vi "Stream LLP Packets to Disk New.vi"(0 "fpga interface in":refnum<k20>, 1 "bytes acquired indicator ref":refnum<vi>, 5 "serial input channel":string, 7 "base packet file path":path, 9 "fetch size (elements)":u32=40960, 11 "error in (no error)":errorcluster, 12 "fetch timeout (s)":dbl=1.0, 13 "log to disk":bool=TRUE) -> (4 "fpga interface out":refnum<k20>, 6 "file path out":path, 8 "acquisition error":bool, 15 "error out":errorcluster)   [LabVIEW 2026]
uses:
  Types/148x_Acq_FPGA_Reference.ctl
  0829f115-c11d-4785-86b3-38f743f517d6.vi
  <vilib>/rvi/errors/niLvFpgaAdjustHostInterfaceError.vi
  <vilib>/rvi/interface/nirviMethod/nirviMethod.xnode
  <vilib>/rvi/interface/nirviReadWriteControl/nirviReadWriteControl.xnode
  <vilib>/FPGAPlugInAG/Dynamic/niLvFpga_AcquireReadRegionFifo_Dynamic.vi
  <vilib>/rvi/errors/niLvFpgaMergeErrorWithErrorCode.vi
  <instrlib>/FlexRIO/Automotive Vision Utility/v1/Host/Automotive Vision Utility.lvlib
  GettingStarted_Acq_148X_Host.lvlib
  Common/GettingStarted_Common_148X_Host.lvlib
  NiFpgaLv.dll
  <vilib>/rvi/interface/Simulation/niFpgaSimulationCallBeginRW.vi
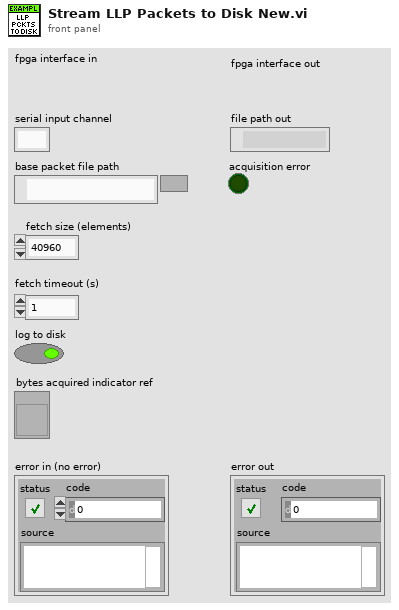
[diagram p1: front panel]
types:
  T1 = typedef "Automotive Vision Utility.lvlib/Serial Channel Type.ctl" = enum16{"Serial Input Channel", "Serial Output Channel", "Unknown Channel Type"}
  T2 = typedef "GettingStarted_Acq_148X_Host.lvlib/148x_Acq_FPGA_Reference.ctl" = refnum<k20>
  T3 = cluster{"acq state":enum8{"Idle", "Wait for First Packet Header", "Acquire", "Wait for Last Packet Header", "Wait for End of Last Packet"}, "stop timed out":bool, "bad packet header":bool, "bad packet payload":bool, "bad packet size":bool, "dram status":cluster{"bytes written":u64, "bytes read":u64, "overflow":bool, "partition full":bool, "last byte flushed":bool}}[]
  T4 = cluster{"acq state":enum8{"Idle", "Wait for First Packet Header", "Acquire", "Wait for Last Packet Header", "Wait for End of Last Packet"}, "stop timed out":bool, "bad packet header":bool, "bad packet payload":bool, "bad packet size":bool, "dram status":cluster{"bytes written":u64, "bytes read":u64, "overflow":bool, "partition full":bool, "last byte flushed":bool}}
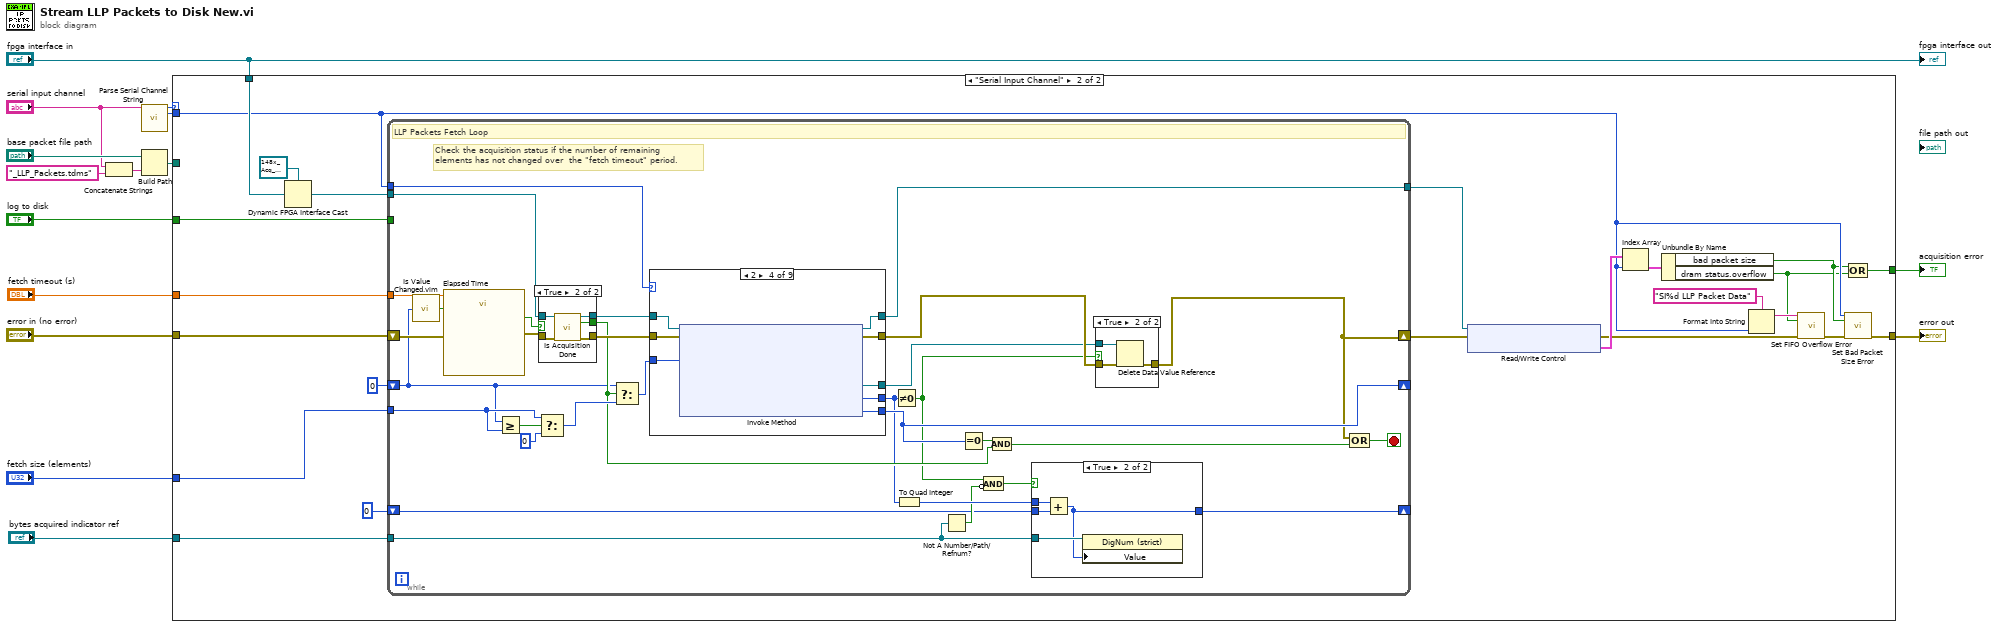
[diagram p0: block diagram]
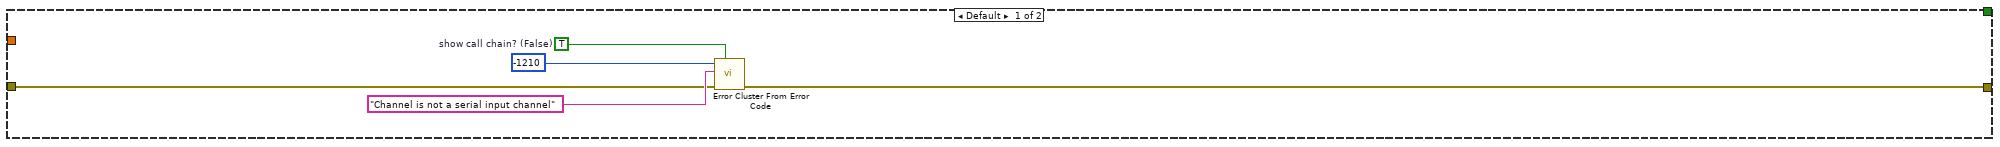
[diagram p2: hidden frame]
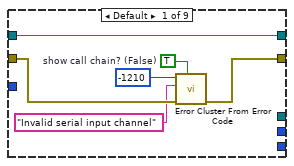
[diagram p6: hidden frame]
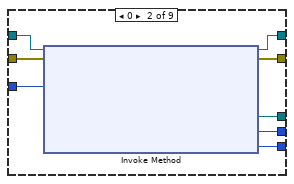
[diagram p7: hidden frame]
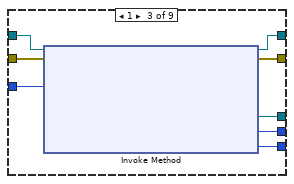
[diagram p8: hidden frame]
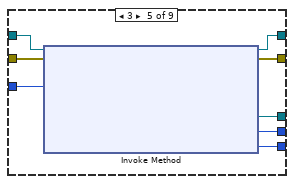
[diagram p9: hidden frame]
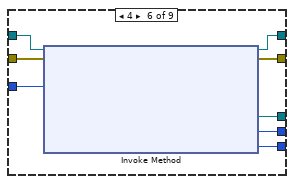
[diagram p10: hidden frame]
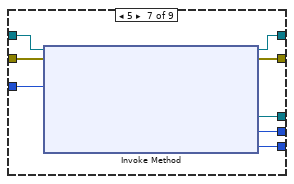
[diagram p11: hidden frame]
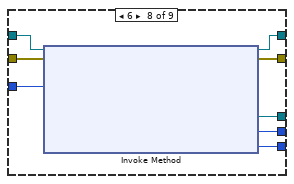
[diagram p12: hidden frame]
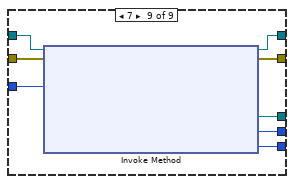
[diagram p13: hidden frame]
diagram:
  n1 = Concatenate Strings("serial input channel", "_LLP_Packets.tdms") -> (w8:string)
  n2 = call <instrlib>:"Parse Serial Channel String.vi"("serial channel string"="serial input channel") -> ("serial channel type"=w11:T1, "channel number"=w12:i32)  [unwired: 13 in]
  n3 = Build Path(base path="base packet file path", name or relative path=w8) -> (appended path=w5:path)
  n4 = case shown="\"Serial Input Channel\"" w11 {
    tunnel: "error in (no error)" -> [w17 w43]
    tunnel: w5 -> [_ _]
    tunnel: [w16 w25] -> w14
    tunnel: [_ w21] -> w13
    tunnel: w12 -> [_ w24]
    tunnel: "fetch size (elements)" -> [_ w40]
    tunnel: "fpga interface in" -> [_ w39]
    tunnel: "fetch timeout (s)" -> [_ w36]
    tunnel: "log to disk" -> [_ w29]
    tunnel: "bytes acquired indicator ref" -> [_ w27]
    frame Default {
      w18 = TRUE  # show call chain? (False)
      n5 = call <vilib>:"Error Cluster From Error Code.vi"("show call chain? (False)"=w18, "error in (no error)"=w17, "error message (\"\")"="Channel is not a serial input channel" ("error message (\"\")"), "error code (0)"=-1210) -> ("error out"=w16:errorcluster)  [unwired: 5 in]
    }
    frame "Serial Input Channel" {
      n6 = Dynamic FPGA Interface Cast(Session In=T2 refnum ("FPGA VI Reference Out"), Type=w39) -> (Session Out=w37:T2)
      n7 = while {
        shift-right: [w54] -> w35
        shift-left: w43 -> [w59]
        tunnel: w37 -> [w63]
        shift-right: [w55] -> _
        shift-left: u32 0 ("Elements Remaining") -> [w56]
        tunnel: [w71] -> w34
        tunnel: w24 -> [w74]
        tunnel: w40 -> [w65]
        tunnel: w36 -> [w70]
        tunnel: w29 -> [_]
        shift-right: [w46] -> _
        shift-left: i64 0 -> [w45]
        tunnel: w27 -> [w47]
        stop <- w75 stop-if-true
        # "Check the acquisition status if the number of remaining \nelements has not changed over  the \"fetch timeout\" period."
        # "LLP Packets Fetch Loop"
        n8 = call "Is Value Changed.vim"("value"=w56) -> ("changed or first call?"=w69:bool)
        n9 = call "Elapsed Time"("Time Target (s)"=w70, "Reset"=w69, "error in (no error)"=w59) -> ("Time has Elapsed"=w61:bool, "error out"=w58:errorcluster)  [unwired: 9 in, 6 out]
        n10 = Greater Or Equal?(x=w56, y=w65) -> (x >= y?=w68:bool)
        n11 = case shown="True" w61 {
          tunnel: w58 -> [w86 w91]
          tunnel: [w86 w90] -> w64
          tunnel: w63 -> [w85 w89]
          tunnel: [w85 w88] -> w62
          tunnel: [_ w87] -> w60
          frame False {
          }
          frame True {
            n12 = call "Is Acquisition Done.vi"("fpga interface in"=w89, "error in (no error)"=w91) -> ("fpga interface out"=w88:T2, "acquisition done"=w87:bool, "error out"=w90:errorcluster)  [unwired: 11 in]
          }
        }
        n13 = Select(t=w65, s=w68, f=u32 0 ("Elements Remaining")) -> (s? t:f=w66:u32)
        n14 = Select(t=w56, s=w60, f=w66) -> (s? t:f=w67:u32)
        n15 = case shown="2" w74 {
          tunnel: w62 -> [w97 w105 w113 w121 w129 w137 w145 w153 w161]
          tunnel: w64 -> [w96 w104 w112 w120 w128 w136 w144 w152 w160]
          tunnel: [_ w103 w111 w119 w127 w135 w143 w151 w159] -> w52
          tunnel: [_ w102 w110 w118 w126 w134 w142 w150 w158] -> w44
          tunnel: w67 -> [_ w101 w109 w117 w125 w133 w141 w149 w157]
          tunnel: [w93 w99 w107 w115 w123 w131 w139 w147 w155] -> w53
          tunnel: [_ w100 w108 w116 w124 w132 w140 w148 w156] -> w55
          tunnel: [w97 w98 w106 w114 w122 w130 w138 w146 w154] -> w71
          frame Default {
            w92 = TRUE  # show call chain? (False)
            n16 = call <vilib>:"Error Cluster From Error Code.vi"("show call chain? (False)"=w92, "error in (no error)"=w96, "error message (\"\")"="Invalid serial input channel" ("error message (\"\")"), "error code (0)"=-1210) -> ("error out"=w93:errorcluster)  [unwired: 5 in]
          }
          frame 0 {
            n17 = xnode "Invoke Method"("FPGA VI Reference In"=w105, "error in"=w104, "Number of Elements"=w101) -> ("FPGA VI Reference Out"=w98:T2, "error out"=w99:errorcluster, "Read Region Reference"=w103:refnum<data-value>, "Elements In Region"=w102:u32, "Elements Remaining"=w100:u32)  [unwired: 1 in]
          }
          frame 1 {
            n18 = xnode "Invoke Method"("FPGA VI Reference In"=w113, "error in"=w112, "Number of Elements"=w109) -> ("FPGA VI Reference Out"=w106:T2, "error out"=w107:errorcluster, "Read Region Reference"=w111:refnum<data-value>, "Elements In Region"=w110:u32, "Elements Remaining"=w108:u32)  [unwired: 1 in]
          }
          frame 2 {
            n19 = xnode "Invoke Method"("FPGA VI Reference In"=w121, "error in"=w120, "Number of Elements"=w117) -> ("FPGA VI Reference Out"=w114:T2, "error out"=w115:errorcluster, "Read Region Reference"=w119:refnum<data-value>, "Elements In Region"=w118:u32, "Elements Remaining"=w116:u32)  [unwired: 1 in]
          }
          frame 3 {
            n20 = xnode "Invoke Method"("FPGA VI Reference In"=w129, "error in"=w128, "Number of Elements"=w125) -> ("FPGA VI Reference Out"=w122:T2, "error out"=w123:errorcluster, "Read Region Reference"=w127:refnum<data-value>, "Elements In Region"=w126:u32, "Elements Remaining"=w124:u32)  [unwired: 1 in]
          }
          frame 4 {
            n21 = xnode "Invoke Method"("FPGA VI Reference In"=w137, "error in"=w136, "Number of Elements"=w133) -> ("FPGA VI Reference Out"=w130:T2, "error out"=w131:errorcluster, "Read Region Reference"=w135:refnum<data-value>, "Elements In Region"=w134:u32, "Elements Remaining"=w132:u32)  [unwired: 1 in]
          }
          frame 5 {
            n22 = xnode "Invoke Method"("FPGA VI Reference In"=w145, "error in"=w144, "Number of Elements"=w141) -> ("FPGA VI Reference Out"=w138:T2, "error out"=w139:errorcluster, "Read Region Reference"=w143:refnum<data-value>, "Elements In Region"=w142:u32, "Elements Remaining"=w140:u32)  [unwired: 1 in]
          }
          frame 6 {
            n23 = xnode "Invoke Method"("FPGA VI Reference In"=w153, "error in"=w152, "Number of Elements"=w149) -> ("FPGA VI Reference Out"=w146:T2, "error out"=w147:errorcluster, "Read Region Reference"=w151:refnum<data-value>, "Elements In Region"=w150:u32, "Elements Remaining"=w148:u32)  [unwired: 1 in]
          }
          frame 7 {
            n24 = xnode "Invoke Method"("FPGA VI Reference In"=w161, "error in"=w160, "Number of Elements"=w157) -> ("FPGA VI Reference Out"=w154:T2, "error out"=w155:errorcluster, "Read Region Reference"=w159:refnum<data-value>, "Elements In Region"=w158:u32, "Elements Remaining"=w156:u32)  [unwired: 1 in]
          }
        }
        n25 = Not Equal To 0?(x=w44) -> (x != 0?=w48:bool)
        n26 = To Quad Integer(1:w44) -> (0:w51:i64)
        n27 = Not A Number/Path/Refnum?(number/path/refnum=w47) -> (NaN/Path/Refnum?=w49:bool)
        n28 = Equal To 0?(x=w55) -> (x = 0?=w57:bool)
        n29 = Compound Arithmetic op=AND(w48, invert w49) -> (w50:bool)
        n30 = Compound Arithmetic op=AND(w57, w60) -> (w72:bool)
        n31 = case shown="True" w50 {
          tunnel: w45 -> [w80 w84]
          tunnel: w51 -> [_ w83]
          tunnel: [w80 w81] -> w46
          tunnel: w47 -> [_ w82]
          frame False {
          }
          frame True {
            n32 = Add(x=w83, y=w84) -> (x+y=w81:i64)
            n33 = property class="DigNum (strict)"(reference=w82, "Value"=w81) -> ()  [unwired: 1 in, 2 out]
          }
        }
        n34 = case shown="True" w48 {
          tunnel: w53 -> [w76 w79]
          tunnel: w52 -> [_ w78]
          tunnel: [w76 w77] -> w54
          frame False {
          }
          frame True {
            n35 = Delete Data Value Reference(data value reference=w78, error in=w79) -> (error out=w77:errorcluster)  [unwired: 1 out]
          }
        }
        n36 = Compound Arithmetic op=OR(w54, w72) -> (w75:bool)
      }
      n37 = xnode "Read/Write Control"("FPGA VI Reference In"=w34, "error in"=w35) -> ("error out"=w32:errorcluster, "serial input channel status"=w33:T3)  [unwired: 1 out]
      n38 = Index Array(array=w33, index=w24) -> (element=w41:T4)
      n39 = Unbundle By Name(w41) -> ("bad packet size"=w23:bool, "dram status.overflow"=w22:bool)
      n40 = Format Into String(format string="SI%d LLP Packet Data" ("fifo name"), w24) -> (resulting string=w31:string)  [unwired: 2 in, 1 out]
      n41 = call "Set FIFO Overflow Error.vi"("fifo name"=w31, "overflow"=w22, "error in (no error)"=w32) -> ("error out"=w26:errorcluster)  [unwired: 12 in]
      n42 = call "Set Bad Packet Size Error.vi"("serial input channel"=w24, "bad packet size"=w23, "error in (no error)"=w26) -> ("error out"=w25:errorcluster)  [unwired: 12 in]
      n43 = Compound Arithmetic op=OR(w23, w22) -> (w21:bool)
    }
  }
  "error out" <- w14
  "acquisition error" <- w13
  "fpga interface out" <- "fpga interface in"
